vi "Stop Core.vi"(10 "final error code":i32, 11 "TDMS Data Logger Actor in":refnum<class "TDMS Data Logger Actor.lvclass">) -> (3 "TDMS Data Logger Actor out":refnum<class "TDMS Data Logger Actor.lvclass">)   [LabVIEW 2024, in "TDMS Data Logger Actor.lvlib" / "TDMS Data Logger Actor.lvclass"]
doc: "<p>(<strong>Filename</strong>: <span class=\"dnl\">Actor Framework.lvlib:Actor.lvclass:Stop Core.vi</span>)</p>\n<p>Defines what the actor does before it stops. Use the <strong>final error code</strong> input to determine whether the actor shut down in response to an error.</p>\n<p>By default, this method passes the Stop message along to all <a href=\"nihelplauncher://docs/csh?context=lvcore_lvcomm_af_launch_nested_actor\">auto-stop nested actors</a>. A descendant class may override this method to define additional behavior, such as shutting down any processes the actor initiated in its override of the <a href=\"nihelplauncher://docs/csh?context=lvcore_lvcomm_af_actor_core\">Actor Core</a> method.</p>"
uses:
  TDMS Data Logger Actor.lvclass
  TDMS Data Logger Actor.lvclass/TDMS Data Logger Actor.ctl
  <vilib>/ActorFramework/Actor/Actor.lvclass
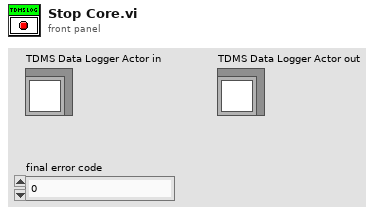
[diagram p1: front panel]
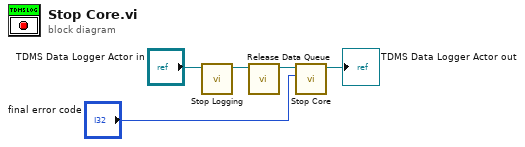
[diagram p0: block diagram]
diagram:
  n1 = call-dynamic "Stop Logging.vi"("Data Logger Interface in"="TDMS Data Logger Actor in") -> ("Data Logger Interface out"=w2:refnum<class "TDMS Data Logger Actor.lvclass">)  [unwired: 9 in, 1 out]
  n2 = call-dynamic "Release Data Queue.vi"("TDMS Data Logger Actor in"=w2) -> ("TDMS Data Logger Actor out"=w1:refnum<class "TDMS Data Logger Actor.lvclass">)  [unwired: 9 in, 1 out]
  n3 = call-parent "Stop Core.vi"("final error code"="final error code", "Actor in"=w1) -> ("Actor out"=→"TDMS Data Logger Actor out":refnum<class "TDMS Data Logger Actor.lvclass">)  [unwired: 9 in]
